vi "Element Events.vi"(8 "error in (no error)":errorcluster, 11 "ButtonControl in":refnum<class "DigitalButtonControl.lvclass">) -> (0 "error out":errorcluster, 2 "Control Events":refnum<class "Control Event Registrations.lvclass">, 3 "ButtonControl out":refnum<class "DigitalButtonControl.lvclass">)   [LabVIEW 2020, in "VolatusGUIElements.lvlib" / "DigitalButtonControl.lvclass"]
uses:
  DigitalButtonControl.lvclass
  C:/dev/lv20CE/relink/lv-volatus/VolatusGUI/GUI Element/GUI Element.lvclass
  C:/dev/lv20CE/relink/lv-volatus/VolatusGUI/OnValueChangeHandler/OnValueChangeHandler.lvclass
  VolatusGUI/Control Event Registrations/Control Event Registrations.lvclass
  VolatusGUI/GUI Element/GUI Element.lvclass/GUI Element.ctl
  DigitalButtonControl.lvclass/DigitalButtonControl.ctl
  VolatusGUI/GUI Element/GUI Element.lvclass
  C:/dev/lv20CE/relink/lv-volatus/VolatusGUIElements/DigitalButtonControl/DigitalButtonControl.lvclass
  C:/dev/lv20CE/relink/lv-volatus/VolatusGUI/OnMouseDown/OnMouseDown.lvclass
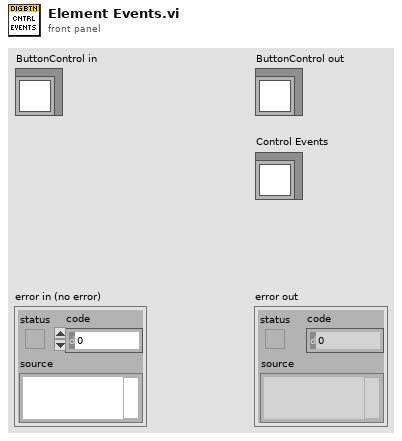
[diagram p1: front panel]
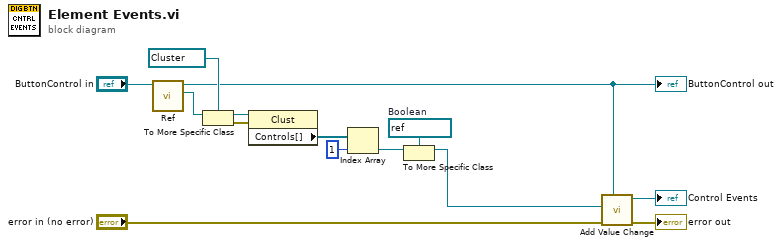
[diagram p0: block diagram]
diagram:
  w7 = refnum<vi> refnum  # Boolean
  n1 = call "Ref.vi"("GUI Element in"="ButtonControl in") -> ("Ref"=w11:refnum<vi>, "GUI Element out"=w2:refnum<class "DigitalButtonControl.lvclass">)  [unwired: 9 in]
  "ButtonControl out" <- w2
  n2 = To More Specific Class(target class=refnum<vi> refnum ("specific class reference"), reference=w11) -> (specific class reference=w9:refnum<vi>, error out=w8:errorcluster)  [unwired: 1 in]
  n3 = property class="Clust"(reference=w9, error in=w8) -> ("Controls[]"=w6:refnum<vi>[])  [unwired: 2 out]
  n4 = Index Array(array=w6, index=1) -> (element=w4:refnum<vi>)
  n5 = To More Specific Class(target class=w7, reference=w4) -> (specific class reference=w1:refnum<vi>)  [unwired: 1 in, 1 out]
  n6 = call "Add Value Change.vi"("Control"=w2, "error in (no error)"="error in (no error)", "CtlRef"=w1) -> ("error out"=→"error out":errorcluster, "Control Event Registrations out"=→"Control Events":refnum<class "Control Event Registrations.lvclass">)  [unwired: 7 in]
